vi "Set configuration chain.vi"(8 "error in (no error)":errorcluster, 9 "class names":string[](array[string]), 10 "configuration":variant[](array[variant]), 11 "Waveform in":refnum<class "Waveform.lvclass">) -> (0 "error out":errorcluster, 3 "Waveform out":refnum<class "Waveform.lvclass">)   [LabVIEW 2012, in "Waveform.lvclass"]
uses:
  Waveform.lvclass
  <vilib>/Distrio/Murmex/Murmex/Murmex.lvclass
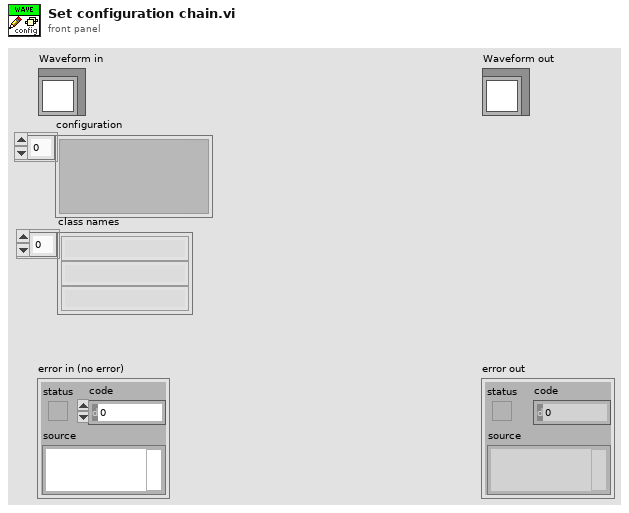
[diagram p1: front panel]
types:
  T1 = typedef "Waveform.lvclass/configuration.ctl" = cluster{"Counter":T2, "analog out":T3, "related components":T4}
  T2 = typedef "Waveform.lvclass/counter_config.ctl" = cluster{"Counter 1":cluster{"Duty cycle":dbl, "Frequency":dbl, "Counter":tag, "Output Terminal":tag}, "Counter 2":cluster{"Duty cycle":dbl, "Frequency":dbl, "Counter":tag, "Output Terminal":tag}}
  T3 = typedef "Waveform.lvclass/AO_config.ctl" = cluster{"AO0":cluster{"min Voltage":dbl, "max Voltage":dbl, "Physical Channel":tag, "trigger edge":i32, "trigger source":tag}, "AO1":cluster{"min Voltage":dbl, "max Voltage":dbl, "Physical Channel":tag, "trigger edge":i32, "trigger source":tag}, "AO2":cluster{"min Voltage":dbl, "max Voltage":dbl, "Physical Channel":tag, "trigger edge":i32, "trigger source":tag}}
  T4 = typedef "Waveform.lvclass/related components.ctl" = cluster{"Camera 1":string, "Camera 2":string, "Camera 3":string}
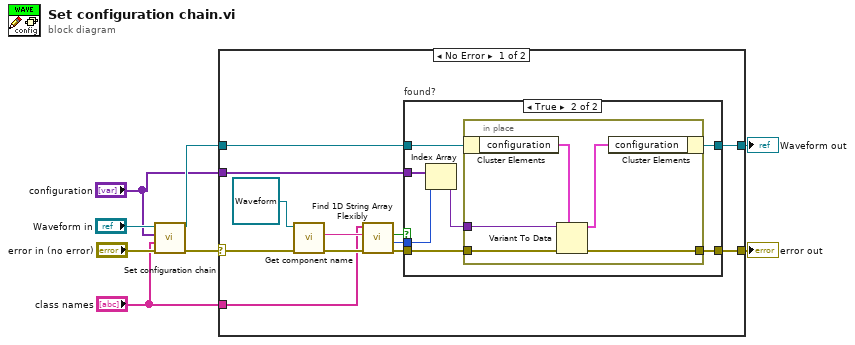
[diagram p0: block diagram]
diagram:
  n1 = call-parent "Set configuration chain.vi"("error in (no error)"="error in (no error)", "class names"="class names", "configuration"="configuration", "Murmex in"="Waveform in") -> ("error out"=w6:errorcluster, "Murmex out"=w4:refnum<class "Waveform.lvclass">)  [unwired: 6 in]
  n2 = case shown="No Error" w6 {
    selector: w6 -> [w18 w36]
    tunnel: [w9 w36] -> w5
    tunnel: w4 -> [w13 w35]
    tunnel: [w10 w35] -> w3
    tunnel: "class names" -> [w16 _]
    tunnel: "configuration" -> [w14 _]
    frame No Error {
      n3 = call <vilib>:"Get component name.vi"("error in (no error)"=w18, "Murmex in"=refnum<class "Waveform.lvclass"> refnum ("Waveform")) -> ("error out"=w20:errorcluster, "component name"=w19:string)  [unwired: 7 in, 1 out]
      n4 = call <vilib>:"Find 1D String Array Flexibly.vi"("error in (no error)"=w20, "element"=w19, "array"=w16) -> ("error out"=w15:errorcluster, "index of element"=w12:i32, "found?"=w11:bool)  [unwired: 6 in]
      n5 = case "found?" shown="True" w11 {
        tunnel: w12 -> [_ w28]
        tunnel: w15 -> [w22 w27]
        tunnel: [w22 w26] -> w9
        tunnel: [w21 w24] -> w10
        tunnel: w14 -> [_ w29]
        tunnel: w13 -> [w21 w23]
        frame False {
        }
        frame True {
          n6 = Index Array(array=w29, index=w28) -> (element=w25:variant)
          n7 = in-place {
            in-place-border: w27 -> [w34]
            in-place-border: [w33] -> w26
            in-place-border: w25 -> [w30]
            n8 = in-place-cluster #1(w23) -> ("configuration"=w32:T1)
            n9 = Variant To Data(error in=w34, type=w32, Variant=w30) -> (data=w31:T1, error out=w33:errorcluster)
            n10 = in-place-cluster #1("configuration"=w31) -> (w24:refnum<class "Waveform.lvclass">)
          }
        }
      }
    }
    frame Error {
    }
  }
  "error out" <- w5
  "Waveform out" <- w3
